vi "RadiogramProcessing.vi"(2 "FileName":string) -> (0 "RTGDataPack":T1)   [LabVIEW 2014]
uses:
  DataTypes/DataTypes.llb/RTG.ctl
  <vilib>/vision/Image Controls.llb/IMAQ Image.ctl
  <vilib>/vision/NI_Vision_Development_Module.lvlib
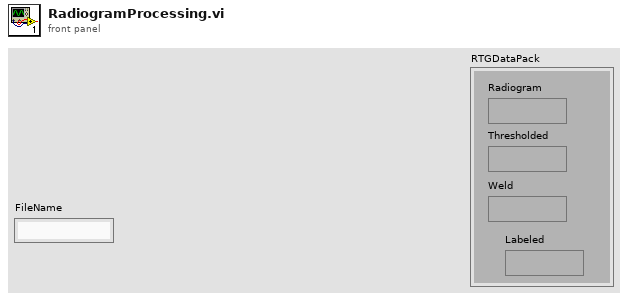
[diagram p1: front panel]
types:
  T1 = typedef "RTG.ctl" = cluster{"Radiogram":T2, "Thresholded":T2, "Weld":T2, "Labeled":T2}
  T2 = typedef "IMAQ Image.ctl" = refnum<image>
  T3 = typedef "Image Type" = u32
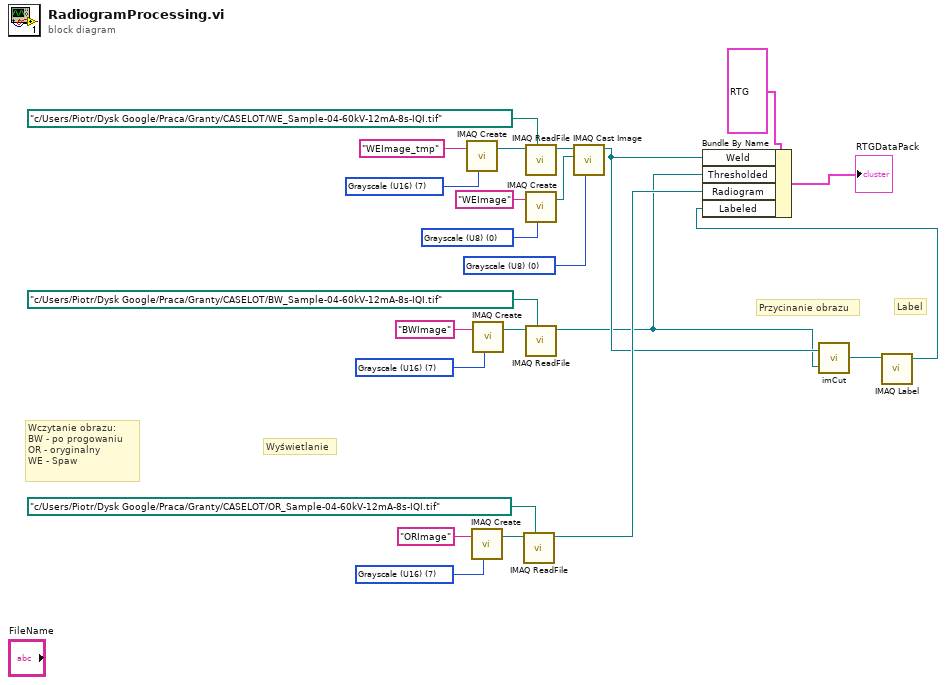
[diagram p0: block diagram]
diagram:
  w9 = T3 0 items=["Grayscale (U8)", "Grayscale (I16)", "Grayscale (SGL)", "Complex (CSG)", "RGB (U32)", "HSL (U32)", "RGB (U64)", "Grayscale (U16)"] ("Image Type")
  w11 = T3 0 items=["Grayscale (U8)", "Grayscale (I16)", "Grayscale (SGL)", "Complex (CSG)", "RGB (U32)", "HSL (U32)", "RGB (U64)", "Grayscale (U16)"] ("Image Type")
  w15 = T3 7 items=["Grayscale (U8)", "Grayscale (I16)", "Grayscale (SGL)", "Complex (CSG)", "RGB (U32)", "HSL (U32)", "RGB (U64)", "Grayscale (U16)"] ("Image Type")
  w19 = T3 7 items=["Grayscale (U8)", "Grayscale (I16)", "Grayscale (SGL)", "Complex (CSG)", "RGB (U32)", "HSL (U32)", "RGB (U64)", "Grayscale (U16)"] ("Image Type")
  w23 = T3 7 items=["Grayscale (U8)", "Grayscale (I16)", "Grayscale (SGL)", "Complex (CSG)", "RGB (U32)", "HSL (U32)", "RGB (U64)", "Grayscale (U16)"] ("Image Type")
  # "Label"
  # "Przycinanie obrazu"
  # "Wczytanie obrazu:\nBW - po progowaniu\nOR - oryginalny\nWE - Spaw"
  # "Wyświetlanie"
  n1 = call "IMAQ Create"("Image Name"="WEImage_tmp", "Image Type"=w15) -> ("New Image"=w12:T2)  [unwired: 3 in, 1 out]
  n2 = call "IMAQ Create"("Image Name"="ORImage", "Image Type"=w19) -> ("New Image"=w18:T2)  [unwired: 3 in, 1 out]
  n3 = call "IMAQ Create"("Image Name"="BWImage", "Image Type"=w23) -> ("New Image"=w22:T2)  [unwired: 3 in, 1 out]
  n4 = call "IMAQ ReadFile"("File Path"=path "c:/Users/Piotr/Dysk Google/Praca/Granty/CASELOT/OR_Sample-04-60kV-12mA-8s-IQI.tif", "Image"=w18) -> ("Image Out"=w6:T2)  [unwired: 5 in, 4 out]
  n5 = call "IMAQ ReadFile"("File Path"=path "c:/Users/Piotr/Dysk Google/Praca/Granty/CASELOT/WE_Sample-04-60kV-12mA-8s-IQI.tif", "Image"=w12) -> ("Image Out"=w13:T2)  [unwired: 5 in, 4 out]
  n6 = call "IMAQ Create"("Image Name"="WEImage", "Image Type"=w9) -> ("New Image"=w8:T2)  [unwired: 3 in, 1 out]
  n7 = call "IMAQ ReadFile"("File Path"=path "c:/Users/Piotr/Dysk Google/Praca/Granty/CASELOT/BW_Sample-04-60kV-12mA-8s-IQI.tif", "Image"=w22) -> ("Image Out"=w2:T2)  [unwired: 5 in, 4 out]
  n8 = call "IMAQ Cast Image"("Image Type"=w11, "Image Dst"=w8, "Image Src"=w13) -> ("Image Dst Out"=w3:T2)  [unwired: 7 in, 1 out]
  n9 = call "imCut.vi"("Image Src"=w2, "Image Mask"=w3) -> ("Image Out"=w4:T2)
  n10 = call "IMAQ Label"("Image Src"=w4) -> ("Image Dst Out"=w1:T2)  [unwired: 3 in, 2 out]
  n11 = Bundle By Name(cluster=T1 {"Radiogram"=refnum, "Thresholded"=refnum, "Weld"=refnum, "Labeled"=refnum} ("RTGDataPack"), "Weld"=w3, "Thresholded"=w2, "Radiogram"=w6, "Labeled"=w1) -> (→"RTGDataPack":T1)
